vi "sCOMS OG TTL.vi"(11 "DataIn":waveform(dbl)) -> (3 "Out":waveform(dbl))   [LabVIEW 2018]
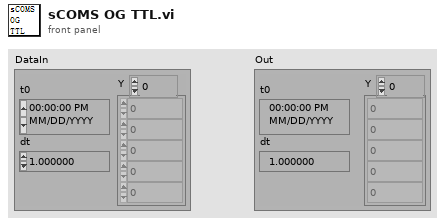
[diagram p1: front panel]
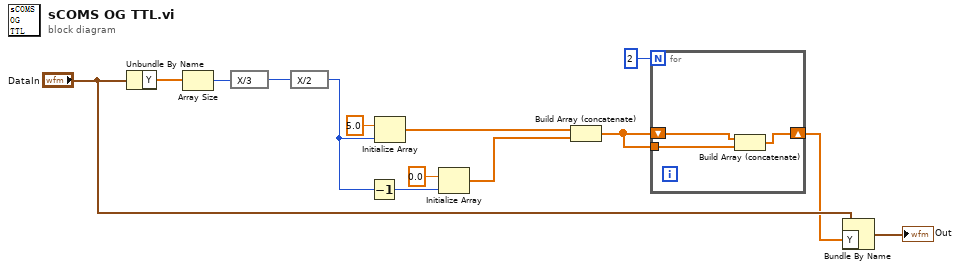
[diagram p0: block diagram]
diagram:
  n1 = Unbundle By Name("DataIn") -> ("Y"=w5:dbl[])
  n2 = Array Size(array=w5) -> (size(s)=w4:i32)
  n3 = expression code="X/3"(w4) -> (w8:i32)
  n4 = expression code="X/2"(w8) -> (w2:i32)
  n5 = Decrement(x=w2) -> (x-1=w1:i32)
  n6 = Initialize Array(5.0 ("element"), w2) -> (w12:dbl[])
  n7 = Initialize Array(0.0 ("element"), w1) -> (w6:dbl[])
  n8 = Build Array (concatenate)(w12, w6) -> (w10:dbl[])
  n9 = for {
    N: 2 -> [_]
    shift-right: [w17] -> w3
    shift-left: w10 -> [w16]
    tunnel: w10 -> [w15]
    n10 = Build Array (concatenate)(w16, w15) -> (w17:dbl[])
  }
  n11 = Bundle By Name(cluster="DataIn", "Y"=w3) -> (→"Out":waveform(dbl))
